vi "DAQmxTaskContainerAcceleratorShutter-Com-Exec.vi"(8 "error in (no error)":errorcluster, 9 "data":variant, 10 "ControlQueue":refnum<queue>, 11 "DAQmxTaskContainer in":refnum<class "DAQmxTaskContainer.lvclass">) -> (0 "error out":errorcluster, 3 "DAQmxTaskContainer out":refnum<class "DAQmxTaskContainer.lvclass">)   [LabVIEW 2015, in "DAQmxTaskContainer.lvclass"]
uses:
  DAQmxTaskContainer.lvclass
  dependecies/ControlsVIs/Clusters-def/ProtypeCommand-DAQmxReply.ctl
  dependecies/ControlsVIs/Clusters-def/SERVER-Commands.ctl
  DAQmxTask.lvclass
  Control/Control-Server/Control-Server.lvclass
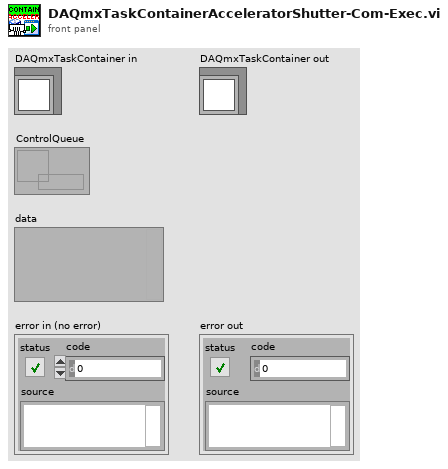
[diagram p1: front panel]
types:
  T1 = typedef "Control-Server.lvclass/SERVER-Commands.ctl" = string
  T2 = typedef "ProtypeCommand-DAQmxReply.ctl" = cluster{"On/Off":bool, "error out":errorcluster}
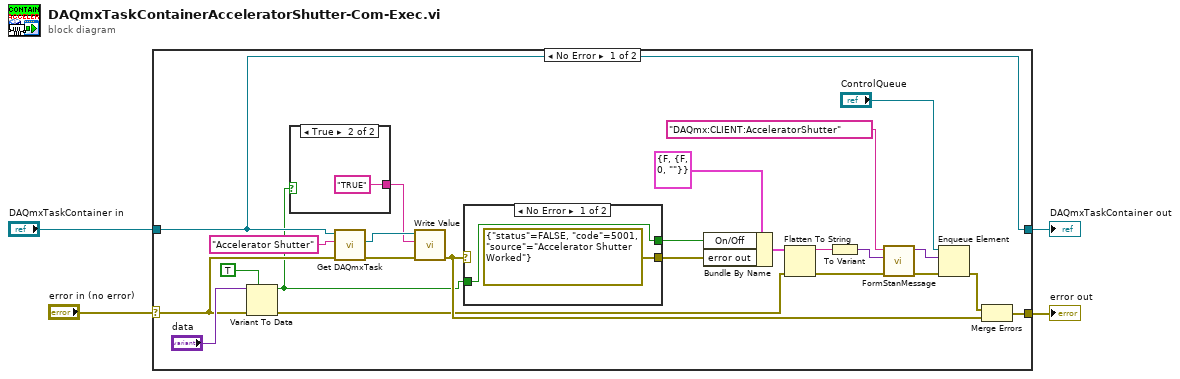
[diagram p0: block diagram]
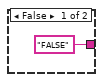
[diagram p2: hidden frame]
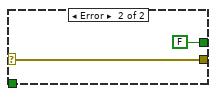
[diagram p3: hidden frame]
diagram:
  n1 = case shown="No Error" "error in (no error)" {
    selector: "error in (no error)" -> [w24 w36]
    tunnel: [w27 w35] -> w4
    tunnel: "DAQmxTaskContainer in" -> [w27 w35]
    tunnel: [w26 w36] -> w2
    frame No Error {
      n2 = Variant To Data(error in=w24, type=TRUE, Variant="data") -> (data=w14:bool, error out=w11:errorcluster)
      n3 = case shown="True" w14 {
        tunnel: ["FALSE" ("Data") "TRUE" ("Data")] -> w19
        frame False {
        }
        frame True {
        }
      }
      n4 = call "Get DAQmxTask.vi"("error in (no error)"=w24, "Task name"="Accelerator Shutter", "DAQmxTaskContainer in"=w27) -> ("error out"=w22:errorcluster, "DAQmx Task"=w20:refnum<class "DAQmxTask.lvclass">)  [unwired: 6 in, 1 out]
      n5 = call-dynamic "Write Value.vi"("error in (no error)"=w22, "Data"=w19, "DAQmxTask en entrée"=w20) -> ("error out"=w18:errorcluster)  [unwired: 7 in, 1 out]
      n6 = case shown="No Error" w18 {
        selector: w18 -> [_ w34]
        tunnel: [errorcluster {"status"=FALSE, "code"=5001, "source"="Accelerator Shutter Worked"} ("error constant") w34] -> w16
        tunnel: [w31 FALSE] -> w15
        tunnel: w14 -> [w31 _]
        frame No Error {
        }
        frame Error {
        }
      }
      n7 = Bundle By Name(cluster=T2 {"On/Off"=FALSE, "error out"={"status"=FALSE, "code"=0, "source"=""}} ("output cluster"), "On/Off"=w15, "error out"=w16) -> (w12:T2)
      n8 = Flatten To String(anything=w12, error in (no error)=w11) -> (data string=w13:string, error out=w8:errorcluster)  [unwired: 2 in, 1 out]
      n9 = To Variant(anything=w13) -> (Variant=w9:variant)
      n10 = call "FormStanMessage.vi"("error in"=w8, "data"=w9, "Command"=T1 "DAQmx:CLIENT:AcceleratorShutter" ("Commands")) -> ("error out"=w6:errorcluster, "message"=w5:variant)  [unwired: 7 in]
      n11 = Enqueue Element(queue="ControlQueue", element=w5, error in (no error)=w6) -> (error out=w10:errorcluster)  [unwired: 1 in, 2 out]
      n12 = Merge Errors(w10, w18) -> (w26:errorcluster)
    }
    frame Error {
    }
  }
  "DAQmxTaskContainer out" <- w4
  "error out" <- w2
